vi "DAQmx Task to VISA Resource.vi"(3 "error in (no error)":errorcluster, 4 "task out":refnum<k21>) -> (0 "error out":errorcluster, 1 "VISAName":string)   [LabVIEW 2020]
uses:
  DAQtoVISA.dll
  <resource>/objmgr/daqmx.rc
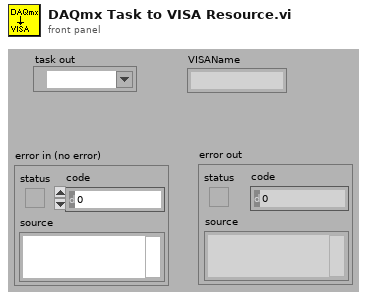
[diagram p1: front panel]
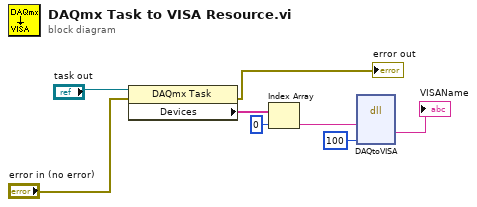
[diagram p0: block diagram]
diagram:
  n1 = property class="DAQmx Task"(reference="task out", error in="error in (no error)") -> (error out=→"error out":errorcluster, "Devices"=w6:tag[])  [unwired: 1 out]
  n2 = Index Array(array=w6, index=0) -> (element=w8:tag)
  n3 = dll-call lib="D:/Development/epl-vi-lib/PXI DAQ VIs/DAQ Engine VIs/AO Gain and Multiplier VIs/DAQtoVISA.dll" fn="DAQtoVISA"("DAQmxName"=w8, "len"=100) -> ("VISAName"=→"VISAName":string)  [unwired: 7 in, 2 out]
